vi "mobileyelanepaser2.vi"() -> (3 "update":bool)   [LabVIEW 2012]
uses:
  G_LCM.vi
  G_SEN.vi
panel:
  in  "path_gain":dbl=0.95
  out "appended array 3":dbl[](array[numeric])
  in  "q_cut":dbl=0.5
  in  "c_cut":dbl=1.0
  in  "b_cut":dbl=0.1
  in  "a_cut":dbl=0.01
  out "lane_old":dbl[](array[numeric])
  out "appended array 2":bool[](array[boolean])
  out "appended array":dbl[](array[numeric])
  in  "gain":dbl=1.0
  out "dt2":dbl
  out "dt":i64
  out "count":u64
  out "lane_empty":dbl[](array[numeric])
  out "Lane_R_M":dbl[](array[numeric])=[0.8601491478953653, 0.8717844136967624, 0.882947592858927, 0.8936326403234123, 0.9038337699485205, 0.9135454576426009, 0.9227624443554423, 0.9314797389261423, 0.9396926207859084, 0.9473966425143293, 0.9545876322477319, 0.9612616959383189, 0.9674152194628639, 0.9730448705798238, 0.9781476007338057, 0.9827206467064133, 0.9867615321125792, 0.9902680687415704, 0.993238357741943, 0.9956707906498045, 0.9975640502598242, 0.9989171113385246, 0.9997292411794617, 1.0, 0.9997292411794617, 0.9989171113385246, 0.9975640502598242, 0.9956707906498045, 0.993238357741943, 0.9902680687415704, 0.9867615321125792, 0.9827206467064133]
  out "Lane_L_M":dbl[](array[numeric])=[0.8601491478953653, 0.8717844136967624, 0.882947592858927, 0.8936326403234123, 0.9038337699485205, 0.9135454576426009, 0.9227624443554423, 0.9314797389261423, 0.9396926207859084, 0.9473966425143293, 0.9545876322477319, 0.9612616959383189, 0.9674152194628639, 0.9730448705798238, 0.9781476007338057, 0.9827206467064133, 0.9867615321125792, 0.9902680687415704, 0.993238357741943, 0.9956707906498045, 0.9975640502598242, 0.9989171113385246, 0.9997292411794617, 1.0, 0.9997292411794617, 0.9989171113385246, 0.9975640502598242, 0.9956707906498045, 0.993238357741943, 0.9902680687415704, 0.9867615321125792, 0.9827206467064133]
  out "r":dbl
  in  "shift_c":dbl=-0.1
  in  "bias_b":dbl=0.005
  out "a":dbl
  out "b":dbl
  out "cl":dbl
  out "cr":dbl
  out "confidance_L":u8
  out "confidance_R":u8
  in  "bias_c":dbl=0.8
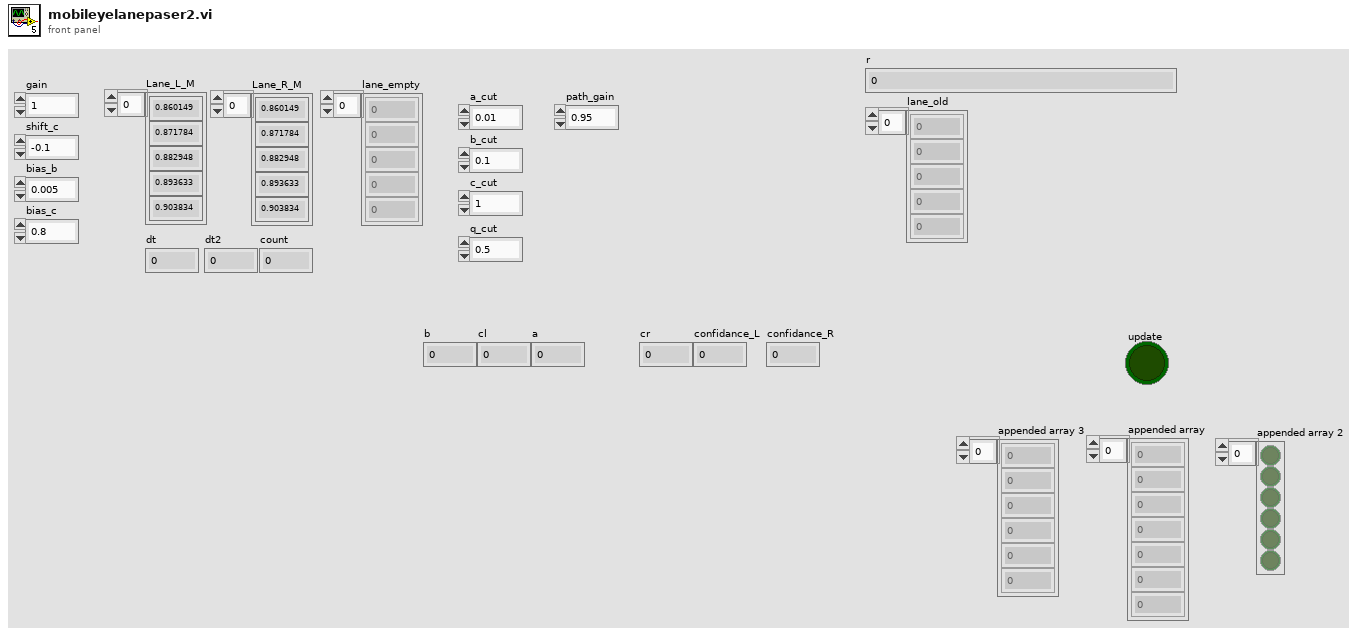
[diagram p1: front panel]
types:
  T1 = cluster{"hash":i64, "sys time":i64, "mobileye":u8[]}
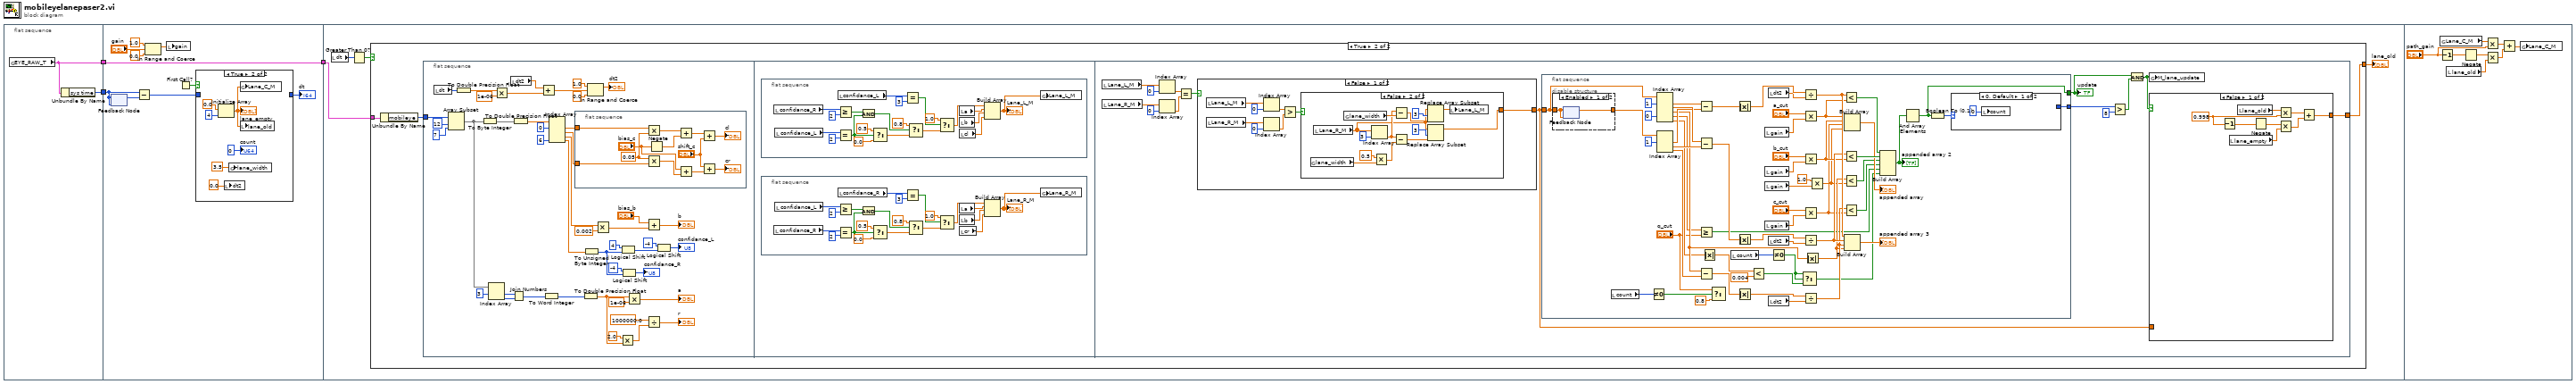
[diagram p0: block diagram]
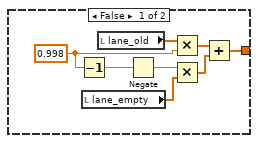
[diagram p3: hidden frame]
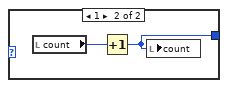
[diagram p4: hidden frame]
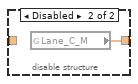
[diagram p5: hidden frame]
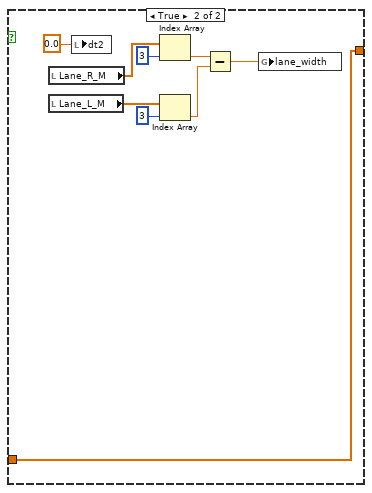
[diagram p6: hidden frame]
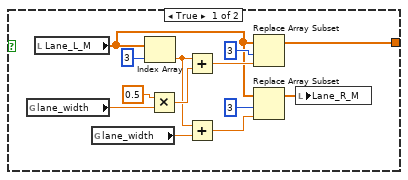
[diagram p7: hidden frame]
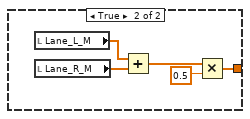
[diagram p8: hidden frame]
diagram:
  n1 = flat-sequence {
    tunnel: [w5] -> w3
    tunnel: [w4] -> w1
    tunnel: w3 -> [w15]
    tunnel: [w15] -> w2
    tunnel: w1 -> [w11]
    tunnel: w2 -> [w26]
    frame #0 {
      n2 = global read "G_LCM.vi" "EYE_RAW_T"() -> (w5:T1)
      n3 = Unbundle By Name(w5) -> ("sys time"=w4:i64)
    }
    frame #1 {
      n4 = feedback #1(w11) -> (w12:i64)
      n5 = feedback-in #1(w11) -> ()
      n6 = Subtract(x=w11, y=w12) -> (x-y=w10:i64)
      n7 = In Range and Coerce(upper limit=1.0, x="gain", lower limit=0.0) -> (coerced(x)=w6:dbl)  [unwired: 1 out]
      n8 = local write "gain"(w6) -> ()
      n9 = First Call?() -> (First Call?: T/F=w14:bool)
      n10 = case shown="True" w14 {
        tunnel: [w16 _] -> w13
        tunnel: w10 -> [w16 _]
        frame False {
        }
        frame True {
          n11 = Initialize Array(0.0 ("element"), 4 ("dimension size")) -> (w17:dbl[])
          "lane_empty" <- w17
          n12 = local write "dt2"(0.0 ("dt2")) -> ()
          n13 = global write "G_SEN.vi" "lane_width"(3.5 ("lane_width")) -> ()
          n14 = global write "G_SEN.vi" "Lane_C_M"(w17) -> ()
          n15 = local write "lane_old"(w17) -> ()
          "count" <- u64 0
        }
      }
      "dt" <- w13
    }
    frame #2 {
      n16 = local read "dt"() -> (w25:i64)
      n17 = Greater Than 0?(x=w25) -> (x > 0?=w24:bool)
      n18 = case shown="True" w24 {
        tunnel: w26 -> [_ w36]
        tunnel: [w27 w35] -> w23
        frame False {
          w29 = 0.998
          n19 = Decrement(x=w29) -> (x-1=w31:dbl)
          n20 = local read "lane_empty"() -> (w28:dbl[])
          n21 = local read "lane_old"() -> (w30:dbl[])
          n22 = Negate(x=w31) -> (-x=w32:dbl)
          n23 = Multiply(x=w30, y=w29) -> (x*y=w33:dbl[])
          n24 = Multiply(x=w32, y=w28) -> (x*y=w34:dbl[])
          n25 = Add(x=w33, y=w34) -> (x+y=w27:dbl[])
        }
        frame True {
          n26 = Unbundle By Name(w36) -> ("mobileye"=w37:u8[])
          n27 = flat-sequence {
            tunnel: w37 -> [w59]
            tunnel: [w141] -> w35
            frame #0 {
              n28 = local read "dt"() -> (w46:i64)
              n29 = Array Subset(array=w59, index=12, length=7) -> (w58:u8[])
              n30 = To Double Precision Float(number=w46) -> (double precision float=w45:dbl)
              n31 = To Byte Integer(number=w58) -> (8bit integer=w78:i8[])
              n32 = Index Array(array=w58, index #1=3 ("index")) -> (element #1=w72:u8, element #2=w71:u8)  [unwired: 1 in]
              n33 = Multiply(x=w45, y=1e-06) -> (x*y=w43:dbl)
              n34 = local read "dt2"() -> (w42:dbl)
              n35 = Join Numbers(hi=w72, lo=w71) -> ((hi.lo)=w70:u16)
              n36 = To Double Precision Float(number=w78) -> (double precision float=w77:dbl[])
              n37 = Add(x=w42, y=w43) -> (x+y=w41:dbl)
              n38 = To Word Integer(number=w70) -> (16bit integer=w69:i16)
              n39 = Index Array(array=w77, index #1=0 ("index"), index #4=6 ("index")) -> (element #1=w76:dbl, element #2=w75:dbl, element #3=w74:dbl, element #4=w65:dbl)  [unwired: 2 in]
              n40 = flat-sequence {
                tunnel: w76 -> [w93]
                tunnel: w75 -> [w92]
                frame #0 {
                  w91 = 0.05 ("y")
                  n41 = Multiply(x=w93, y=w91) -> (x*y=w89:dbl)
                  n42 = Multiply(x=w91, y=w92) -> (x*y=w90:dbl)
                  n43 = Negate(x="bias_c") -> (-x=w87:dbl)
                  n44 = Add(x=w89, y=w87) -> (x+y=w86:dbl)
                  n45 = Add(x="bias_c", y=w90) -> (x+y=w84:dbl)
                  n46 = Add(x=w86, y="shift_c") -> (x+y=→"cl":dbl)
                  n47 = Add(x="shift_c", y=w84) -> (x+y=→"cr":dbl)
                }
              }
              n48 = To Double Precision Float(number=w69) -> (double precision float=w47:dbl)
              n49 = To Unsigned Byte Integer(number=w65) -> (unsigned 8bit integer=w63:u8)
              n50 = In Range and Coerce(upper limit=1.0, x=w41, lower limit=0.0) -> (coerced(x)=→"dt2":dbl)  [unwired: 1 out]
              n51 = Multiply(x=w74, y=0.002) -> (x*y=w55:dbl)
              n52 = Logical Shift(y=i16 4, x=w63) -> (x << y=w61:u8)
              n53 = Multiply(x=2.0, y=w47) -> (x*y=w50:dbl)
              n54 = Logical Shift(y=i16 -4, x=w63) -> (x << y=→"confidance_R":u8)
              n55 = Multiply(x=w47, y=1e-06) -> (x*y=→"a":dbl)
              n56 = Add(x="bias_b", y=w55) -> (x+y=→"b":dbl)
              n57 = Divide(x=1000000.0 ("y"), y=w50) -> (x/y=→"r":dbl)
              n58 = Logical Shift(y=i16 -4, x=w61) -> (x << y=→"confidance_L":u8)
            }
            frame #1 {
              n59 = flat-sequence {
                frame #0 {
                  n60 = local read "confidance_R"() -> (w134:u8)
                  n61 = local read "confidance_L"() -> (w122:u8)
                  n62 = Greater Or Equal?(x=w134, y=u8 2) -> (x >= y?=w117:bool)
                  n63 = Equal?(x=w122, y=u8 2) -> (x = y?=w116:bool)
                  n64 = local read "confidance_L"() -> (w132:u8)
                  n65 = And(x=w117, y=w116) -> (x .and. y?=w125:bool)
                  n66 = Select(t=0.5, s=w116, f=0.0) -> (s? t:f=w119:dbl)
                  n67 = Equal?(x=w132, y=u8 3) -> (x = y?=w126:bool)
                  n68 = Select(t=0.8, s=w125, f=w119) -> (s? t:f=w123:dbl)
                  n69 = Select(t=1.0, s=w126, f=w123) -> (s? t:f=w128:dbl)
                  n70 = local read "a"() -> (w129:dbl)
                  n71 = local read "b"() -> (w130:dbl)
                  n72 = local read "cl"() -> (w131:dbl)
                  n73 = Build Array(w128, w129, w130, w131) -> (w115:dbl[])
                  "Lane_L_M" <- w115
                  n74 = global write "G_SEN.vi" "Lane_L_M"(w115) -> ()
                }
              }
              n75 = flat-sequence {
                frame #0 {
                  n76 = local read "confidance_R"() -> (w101:u8)
                  n77 = local read "confidance_L"() -> (w113:u8)
                  n78 = Greater Or Equal?(x=w113, y=u8 2) -> (x >= y?=w96:bool)
                  n79 = Equal?(x=w101, y=u8 2) -> (x = y?=w95:bool)
                  n80 = local read "confidance_R"() -> (w111:u8)
                  n81 = And(x=w96, y=w95) -> (x .and. y?=w104:bool)
                  n82 = Select(t=0.5, s=w95, f=0.0) -> (s? t:f=w98:dbl)
                  n83 = Equal?(x=w111, y=u8 3) -> (x = y?=w106:bool)
                  n84 = Select(t=0.8, s=w104, f=w98) -> (s? t:f=w102:dbl)
                  n85 = Select(t=1.0, s=w106, f=w102) -> (s? t:f=w107:dbl)
                  n86 = local read "a"() -> (w108:dbl)
                  n87 = local read "b"() -> (w109:dbl)
                  n88 = local read "cr"() -> (w110:dbl)
                  n89 = Build Array(w107, w108, w109, w110) -> (w94:dbl[])
                  "Lane_R_M" <- w94
                  n90 = global write "G_SEN.vi" "Lane_R_M"(w94) -> ()
                }
              }
            }
            frame #2 {
              n91 = local read "Lane_L_M"() -> (w142:dbl[])
              n92 = local read "Lane_R_M"() -> (w143:dbl[])
              n93 = Index Array(array=w142, index=0) -> (element=w147:dbl)
              n94 = Index Array(array=w143, index=0) -> (element=w146:dbl)
              n95 = Equal?(x=w147, y=w146) -> (x = y?=w145:bool)
              n96 = case shown="False" w145 {
                tunnel: [w234 w268] -> w144
                frame False {
                  n97 = local read "Lane_L_M"() -> (w232:dbl[])
                  n98 = local read "Lane_R_M"() -> (w233:dbl[])
                  n99 = Index Array(array=w232, index=0) -> (element=w237:dbl)
                  n100 = Index Array(array=w233, index=0) -> (element=w236:dbl)
                  n101 = Greater?(x=w237, y=w236) -> (0:w235:bool)
                  n102 = case shown="False" w235 {
                    tunnel: [w249 w262] -> w234
                    frame True {
                      n103 = global read "G_SEN.vi" "lane_width"() -> (w246:dbl)
                      n104 = local read "Lane_L_M"() -> (w240:dbl[])
                      n105 = global read "G_SEN.vi" "lane_width"() -> (w242:dbl)
                      n106 = Index Array(array=w240, index=3) -> (element=w243:dbl)
                      n107 = Multiply(x=0.5 ("y"), y=w246) -> (x*y=w248:dbl)
                      n108 = Add(x=w243, y=w248) -> (x+y=w251:dbl)
                      n109 = Add(x=w243, y=w242) -> (x+y=w244:dbl)
                      n110 = Replace Array Subset(array=w240, new element=w251, index=3) -> (w249:dbl[])
                      n111 = Replace Array Subset(array=w240, new element=w244, index=3) -> (w241:dbl[])
                      n112 = local write "Lane_R_M"(w241) -> ()
                    }
                    frame False {
                      n113 = global read "G_SEN.vi" "lane_width"() -> (w259:dbl)
                      n114 = local read "Lane_R_M"() -> (w254:dbl[])
                      n115 = global read "G_SEN.vi" "lane_width"() -> (w256:dbl)
                      n116 = Index Array(array=w254, index=3) -> (element=w255:dbl)
                      n117 = Multiply(x=0.5 ("y"), y=w259) -> (x*y=w261:dbl)
                      n118 = Subtract(x=w255, y=w256) -> (x-y=w257:dbl)
                      n119 = Subtract(x=w255, y=w261) -> (x-y=w264:dbl)
                      n120 = Replace Array Subset(array=w254, new element=w257, index=3) -> (w253:dbl[])
                      n121 = Replace Array Subset(array=w254, new element=w264, index=3) -> (w262:dbl[])
                      n122 = local write "Lane_L_M"(w253) -> ()
                    }
                  }
                }
                frame True {
                  n123 = local read "Lane_L_M"() -> (w266:dbl[])
                  n124 = local read "Lane_R_M"() -> (w267:dbl[])
                  n125 = Add(x=w266, y=w267) -> (x+y=w270:dbl[])
                  n126 = Multiply(x=w270, y=0.5) -> (x*y=w268:dbl[])
                }
              }
              n127 = flat-sequence {
                tunnel: w144 -> [w189]
                tunnel: [w163] -> w138
                tunnel: [w162] -> w140
                frame #0 {
                  n128 = disable-structure shown="Enabled" {
                    disable-tunnel: w189 -> [w213 _]
                    disable-tunnel: [w212 w214] -> w188
                    frame Enabled {
                      n129 = feedback #2(w213) -> (w212:dbl[])
                      n130 = feedback-in #2(w213) -> ()
                    }
                    frame Disabled {
                      n131 = global read "G_SEN.vi" "Lane_C_M"() -> (w214:dbl[])
                    }
                  }
                  n132 = local read "count"() -> (w153:u64)
                  n133 = Not Equal To 0?(x=w153) -> (x != 0?=w152:bool)
                  n134 = Index Array(array=w189, index #1=1 ("index"), index #4=0 ("index")) -> (element #1=w196:dbl, element #2=w202:dbl, element #3=w190:dbl, element #4=w174:dbl, element #5=w158:dbl)  [unwired: 3 in]
                  n135 = Index Array(array=w188, index #1=1 ("index")) -> (element #1=w195:dbl, element #2=w201:dbl, element #3=w194:dbl)  [unwired: 2 in]
                  n136 = Subtract(x=w196, y=w195) -> (x-y=w206:dbl)
                  n137 = Subtract(x=w202, y=w201) -> (x-y=w198:dbl)
                  n138 = Greater Or Equal?(x=w174, y="q_cut") -> (x >= y?=w167:bool)
                  n139 = Subtract(x=w190, y=w194) -> (x-y=w191:dbl)
                  n140 = Absolute Value(x=w158) -> (abs(x)=w157:dbl)
                  n141 = Select(t="q_cut", s=w152, f=0.8) -> ()  [unwired: 1 out]
                  n142 = local read "count"() -> (w160:u64)
                  n143 = Absolute Value(x=w206) -> (abs(x)=w205:dbl)
                  n144 = Absolute Value(x=w198) -> (abs(x)=w199:dbl)
                  n145 = Absolute Value(x=w191) -> (abs(x)=w193:dbl)
                  n146 = Less?(x=w157, y=0.004) -> (x < y?=w156:bool)
                  n147 = local read "gain"() -> (w183:dbl)
                  n148 = local read "gain"() -> (w181:dbl)
                  n149 = local read "gain"() -> (w176:dbl)
                  n150 = local read "gain"() -> (w178:dbl)
                  n151 = local read "dt2"() -> (w204:dbl)
                  n152 = local read "dt2"() -> (w200:dbl)
                  n153 = local read "dt2"() -> (w192:dbl)
                  n154 = Not Equal To 0?(x=w160) -> (x != 0?=w159:bool)
                  n155 = Select(t=w159, s=w159, f=w156) -> (s? t:f=w155:bool)
                  n156 = Divide(x=w205, y=w204) -> (x/y=w187:dbl)
                  n157 = Multiply(x="a_cut", y=w183) -> (x*y=w173:dbl)
                  n158 = Multiply(x="b_cut", y=w181) -> (x*y=w172:dbl)
                  n159 = Multiply(x="c_cut", y=w178) -> (x*y=w171:dbl)
                  n160 = Divide(x=w199, y=w200) -> (x/y=w186:dbl)
                  n161 = Divide(x=w193, y=w192) -> (x/y=w185:dbl)
                  n162 = Absolute Value(x=w190) -> (abs(x)=w184:dbl)
                  n163 = Multiply(x=1.0 ("y"), y=w176) -> (x*y=w170:dbl)
                  n164 = Less?(x=w187, y=w173) -> (x < y?=w203:bool)
                  n165 = Less?(x=w186, y=w172) -> (x < y?=w197:bool)
                  n166 = Less?(x=w184, y=w170) -> (x < y?=w166:bool)
                  n167 = Less?(x=w185, y=w171) -> (x < y?=w165:bool)
                  n168 = Build Array(w173, w172, w171, w170) -> (→"appended array":dbl[])
                  n169 = Build Array(w187, w186, w185, w184) -> (→"appended array 3":dbl[])
                  n170 = Build Array(w203, w197, w166, w165, w167, w155) -> (w168:bool[])
                  "appended array 2" <- w168
                  n171 = And Array Elements(Boolean array=w168) -> (logical AND=w163:bool)
                  n172 = Boolean To (0,1)(Boolean=w163) -> (0, 1=w161:i16)
                  n173 = case shown="0, Default" w161 {
                    tunnel: [_ w210] -> w162
                    frame 0, Default {
                      n174 = local write "count"(u64 0 ("count")) -> ()
                    }
                    frame 1 {
                      n175 = local read "count"() -> (w211:u64)
                      n176 = Increment(x=w211) -> (x+1=w210:u64)
                      n177 = local write "count"(w210) -> ()
                    }
                  }
                }
              }
              n178 = Greater?(x=w140, y=u64 8) -> (0:w137:bool)
              n179 = And(x=w138, y=w137) -> (x .and. y?=w136:bool)
              n180 = global write "G_SEN.vi" "M_lane_update"(w136) -> ()
              n181 = case shown="False" w136 {
                tunnel: w144 -> [_ w224]
                tunnel: [w215 w224] -> w141
                frame False {
                  w217 = 0.998
                  n182 = Decrement(x=w217) -> (x-1=w219:dbl)
                  n183 = local read "lane_empty"() -> (w216:dbl[])
                  n184 = local read "lane_old"() -> (w218:dbl[])
                  n185 = Negate(x=w219) -> (-x=w220:dbl)
                  n186 = Multiply(x=w218, y=w217) -> (x*y=w221:dbl[])
                  n187 = Multiply(x=w220, y=w216) -> (x*y=w222:dbl[])
                  n188 = Add(x=w221, y=w222) -> (x+y=w215:dbl[])
                }
                frame True {
                  n189 = local read "Lane_R_M"() -> (w226:dbl[])
                  n190 = local read "Lane_L_M"() -> (w225:dbl[])
                  n191 = local write "dt2"(0.0 ("dt2")) -> ()
                  n192 = Index Array(array=w226, index=3) -> (element=w230:dbl)
                  n193 = Index Array(array=w225, index=3) -> (element=w229:dbl)
                  n194 = Subtract(x=w230, y=w229) -> (x-y=w228:dbl)
                  n195 = global write "G_SEN.vi" "lane_width"(w228) -> ()
                }
              }
              "update" <- w138
            }
          }
        }
      }
      "lane_old" <- w23
    }
    frame #3 {
      n196 = Decrement(x="path_gain") -> (x-1=w276:dbl)
      n197 = global read "G_SEN.vi" "Lane_C_M"() -> (w277:dbl[])
      n198 = local read "lane_old"() -> (w271:dbl[])
      n199 = Negate(x=w276) -> (-x=w275:dbl)
      n200 = Multiply(x=w277, y="path_gain") -> (x*y=w274:dbl[])
      n201 = Multiply(x=w275, y=w271) -> (x*y=w273:dbl[])
      n202 = Add(x=w274, y=w273) -> (x+y=w272:dbl[])
      n203 = global write "G_SEN.vi" "Lane_C_M"(w272) -> ()
    }
  }
